vi "Acknowledge bank data.vi"(8 "error in":errorcluster, 10 "Timeout,s":dbl=10.0, 11 "OPC connections":T1) -> (0 "error out":errorcluster, 3 "OPC connections out":T1, 4 "Data ready":bool)   [LabVIEW 2015]
uses:
  OPC connections.ctl
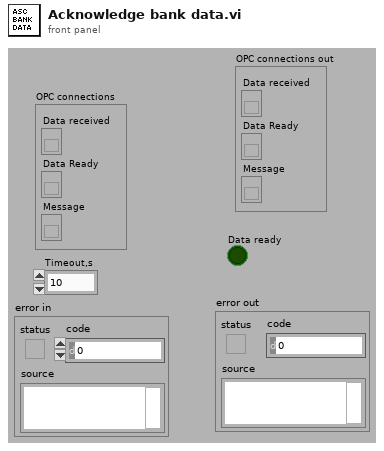
[diagram p1: front panel]
types:
  T1 = typedef "OPC connections.ctl" = cluster{"Data received":refnum<k13>, "Data Ready":refnum<k13>, "Message":refnum<k13>}
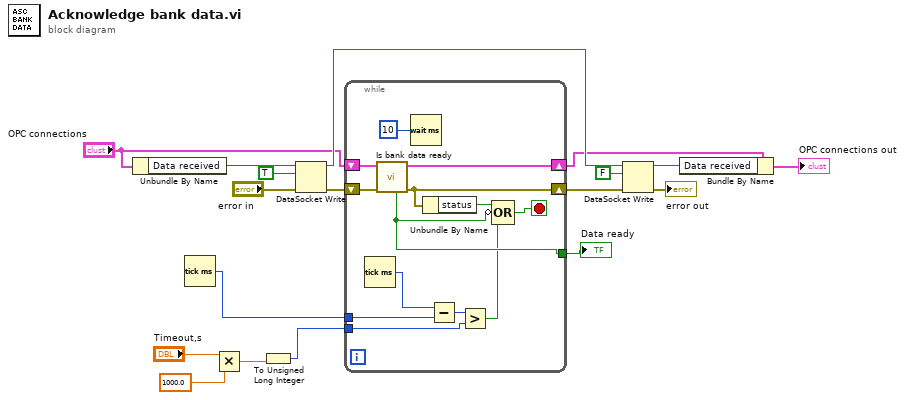
[diagram p0: block diagram]
diagram:
  n1 = Unbundle By Name("OPC connections") -> ("Data received"=w12:refnum<k13>)
  n2 = Tick Count (ms)() -> (millisecond timer value=w5:u32)
  n3 = Multiply(x="Timeout,s", y=1000.0) -> (x*y=w2:dbl)
  n4 = To Unsigned Long Integer(number=w2) -> (unsigned 32bit integer=w1:u32)
  n5 = DataSocket Write(8:"error in", 10:TRUE, 11:w12) -> (0:w14:errorcluster, 3:w17:refnum<k13>)  [unwired: 1 in, 1 out]
  n6 = while {
    shift-right: [w30] -> w15
    shift-left: w14 -> [w31]
    tunnel: [w27] -> w6
    shift-right: [w24] -> w9
    shift-left: "OPC connections" -> [w25]
    tunnel: w5 -> [w22]
    tunnel: w1 -> [w20]
    stop <- w29 stop-if-true
    n7 = Tick Count (ms)() -> (millisecond timer value=w23:u32)
    n8 = call "Is bank data ready.vi"("error IO"=w31, "OPC connections"=w25) -> ("error out"=w30:errorcluster, "OPC connections out"=w24:T1, "Data ready"=w27:bool)  [unwired: 7 in]
    n9 = Wait (ms)(milliseconds to wait=u32 10) -> ()  [unwired: 1 out]
    n10 = Unbundle By Name(w30) -> ("status"=w28:bool)
    n11 = Subtract(x=w23, y=w22) -> (x-y=w21:u32)
    n12 = Greater?(x=w21, y=w20) -> (0:w19:bool)
    n13 = Compound Arithmetic op=OR(w28, invert w27, w19) -> (w29:bool)
  }
  "Data ready" <- w6
  n14 = DataSocket Write(8:w15, 10:FALSE, 11:w17) -> (0:→"error out":errorcluster, 3:w8:refnum<k13>)  [unwired: 1 in, 1 out]
  n15 = Bundle By Name(cluster=w9, "Data received"=w8) -> (→"OPC connections out":T1)
